vi "Begin.vi"(8 "error in":errorcluster) -> (0 "error out":errorcluster)   [LabVIEW 2015]
doc: "Called before other user functions, this VI is expected to open initial I/O refnums, load in file data, and do all program initialization. Notice that the <B>error out</B> terminal is simply used for data flow. Wiring it to other structures or subVIs ensures that this VI runs first."
uses:
  <vilib>/Rock Robotics/WPI/Camera/WPI_CameraImageSize.ctl
  <vilib>/Rock Robotics/WPI/DriverStation/WPI_DriverStationRobotMode2.ctl
  <vilib>/Rock Robotics/WPI/Joystick/WPI_JoystickDeviceEnum.ctl
  <vilib>/Rock Robotics/WPI/Solenoid/WPI_SolenoidChannel.ctl
  <vilib>/Rock Robotics/SystemInterfaces/AI/FPGA_AIChannel.ctl
  <vilib>/Rock Robotics/WPI/CAN/TalonSRX/WPI_CANTalonSRX_BrakeOverride.ctl
  <vilib>/Rock Robotics/SystemInterfaces/DIO/FPGA_DIOChannel.ctl
  <vilib>/Rock Robotics/SystemInterfaces/DIO/FPGA_DIOPWMChannel.ctl
  <vilib>/Rock Robotics/WPI/CAN/TalonSRX/WPI_CANTalonSRX_APIFeedbackSelect.ctl
  <vilib>/Rock Robotics/WPI/CAN/TalonSRX/WPI_CANTalonSRX_StatusFrame.ctl
  <vilib>/Rock Robotics/WPI/AnalogOutput/WPI_AnalogOutputChannel.ctl
  <vilib>/Rock Robotics/SystemInterfaces/spilib/spi_bus.ctl
  Robot Global Data.vi
  <vilib>/Rock Robotics/WPI/Utilities/WPI_GetSetVariantRefNum.vi
  <vilib>/Rock Robotics/WPI/Solenoid/WPI_SolenoidOpenSingle.vi
  <vilib>/Rock Robotics/WPI/MotorControl/WPI_MotorControlOpenCANTalonSRX.vi
  <vilib>/Rock Robotics/WPI/MotorControl/WPI_MotorControlOpen VictorSP.vi
  <vilib>/Rock Robotics/WPI/Counter/WPI_CounterDigitalInputToDigitalSource.vi
  navX.Library.v2/navX Library v2/IO/Open/Z900_navX_Open_SPI.vi
  <vilib>/Rock Robotics/WPI/CAN/TalonSRX/WPI_CANTalonSRX_APIControlMode.ctl
  <vilib>/Rock Robotics/WPI/Camera/WPI_CameraWhite Balance Values.ctl
  <vilib>/Rock Robotics/WPI/Camera/WPI_CameraExposure Values.ctl
  <vilib>/Rock Robotics/WPI/Ultrasonic/WPI_SonarSRF04DigitalOpen.vi
  <vilib>/Rock Robotics/WPI/Ultrasonic/WPI_SonarSRF04DigitalRefNum Registry Set.vi
  navX-MXP Library/navX-MXP IMU.lvlib
  navX-MXP Library/COMMON/TypeDefs/Value TypeDefs/navX Interface Protocol.ctl
  navX-MXP Library/COMMON/TypeDefs/Value TypeDefs/navX Update Rate.ctl
  <vilib>/Rock Robotics/WPI/Camera/WPI_CameraFrameRate.ctl
  navX.Library.v2/navX Library v2/navX Library v2.lvlib
panel:
  in  "Image Size":T1=enum."320x240"
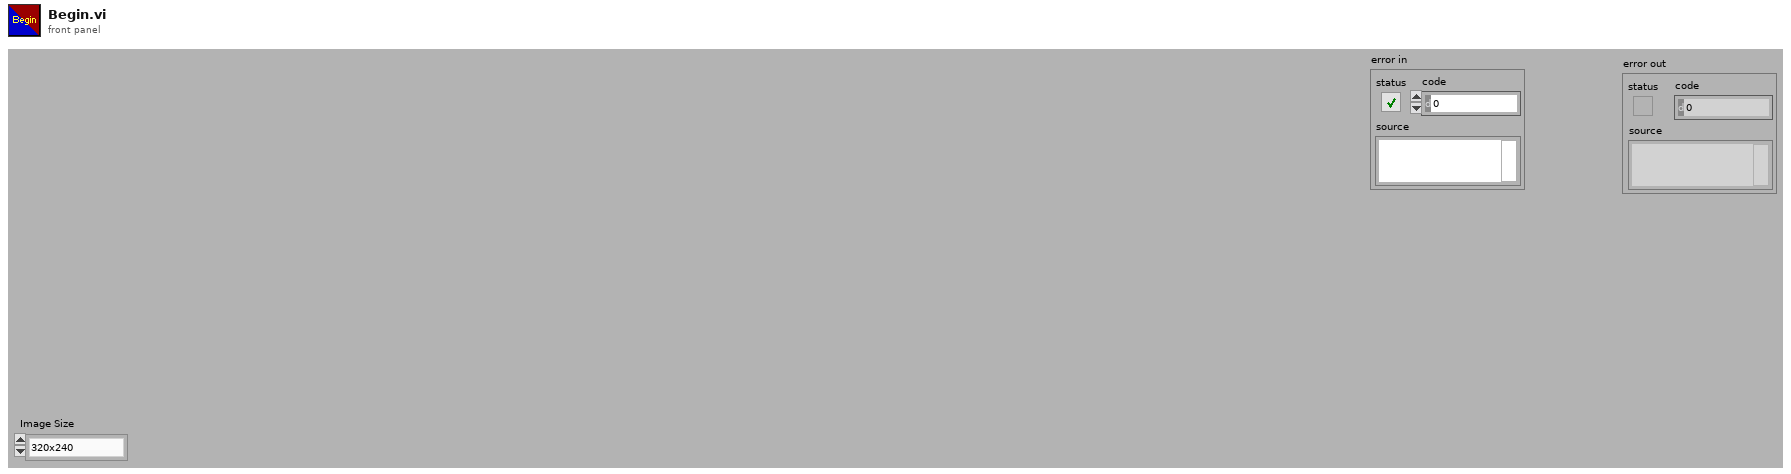
[diagram p1: front panel]
types:
  T1 = typedef "WPI_CameraImageSize.ctl" = enum16{"640x480", "320x240", "160x120", "Custom"}
  T2 = typedef "WPI_AnalogOutputChannel.ctl" = enum8{"AO MXP 0", "AO MXP 1", "Invalid"}
  T3 = typedef "FPGA_AIChannel.ctl" = enum8{"AI 0", "AI 1", "AI 2", "AI 3", "AI MXP 0", "AI MXP 1", "AI MXP 2", "AI MXP 3", "Invalid"}
  T4 = typedef "WPI_CANTalonSRX_StatusFrame.ctl" = enum16{"General Status Frame", "Feedback Status Frame", "Quadrature Status Frame", "Analog Temp Vbat Status Frame", "Pulse Width Status Frame"}
  T5 = typedef "WPI_CANTalonSRX_BrakeOverride.ctl" = enum8{"No Override", "Override to Coast", "Override to Brake"}
  T6 = typedef "WPI_SolenoidChannel.ctl" = enum8{"Solenoid 0", "Solenoid 1", "Solenoid 2", "Solenoid 3", "Solenoid 4", "Solenoid 5", "Solenoid 6", "Solenoid 7", "Invalid"}
  T7 = typedef "WPI_CANTalonSRX_APIFeedbackSelect.ctl" = enum16{"Digital Quadrature Encoder", "Analog Potentiometer", "Analog Encoder", "Count on Quad-A (Rising-Edge)", "Count on Quad-A (Falling-Edge)", "CTR Magnetic Enc (Absolute)", "CTR Magnetic Enc (Relative)", "Pulse Width"}
  T8 = typedef "FPGA_DIOChannel.ctl" = enum8{"DIO 0", "DIO 1", "DIO 2", "DIO 3", "DIO 4", "DIO 5", "DIO 6", "DIO 7", "DIO 8", "DIO 9", "DIO MXP 0", "DIO MXP 1", "DIO MXP 2", "DIO MXP 3", "DIO MXP 4", "DIO MXP 5", "DIO MXP 6", "DIO MXP 7", "DIO MXP 8", "DIO MXP 9", "DIO MXP 10", "DIO MXP 11", "DIO MXP 12", "DIO MXP 13", "DIO MXP 14", "DIO MXP 15", "Invalid"}
  T9 = typedef "FPGA_DIOPWMChannel.ctl" = enum8{"PWM 0", "PWM 1", "PWM 2", "PWM 3", "PWM 4", "PWM 5", "PWM 6", "PWM 7", "PWM 8", "PWM 9", "PWM MXP 0", "PWM MXP 1", "PWM MXP 2", "PWM MXP 3", "PWM MXP 4", "PWM MXP 5", "PWM MXP 6", "PWM MXP 7", "PWM MXP 8", "PWM MXP 9", "Invalid"}
  T10 = typedef "WPI_JoystickDeviceEnum.ctl" = enum16{"USB 0", "USB 1", "USB 2", "USB 3", "USB 4", "USB 5"}
  T11 = typedef "WPI_DriverStationRobotMode2.ctl" = enum16{"Autonomous Disabled", "Autonomous Enabled", "Teleop Disabled", "Teleop Enabled", "Disconnected", "Finish", "Test Disabled", "Test Enabled", "Emergency Stopped"}
  T12 = typedef "navX-MXP IMU.lvlib/navX Update Rate.ctl" = u8
  T13 = typedef "navX-MXP IMU.lvlib/navX Interface Protocol.ctl" = enum16{"SPI", "I2C"}
  T14 = typedef "spi_bus.ctl" = enum16{"SPI On-Board, CS0", "SPI On-Board, CS1", "SPI On-Board, CS2", "SPI On-Board, CS3", "SPI MXP", "Invalid"}
  T15 = typedef "navX-MXP IMU.lvlib/navX Device TypeDef.ctl" = cluster{"navX Interface Protocol":T13, "navX Interface Protocol TypeDefs":cluster{"SPIDevRef":T16, "I2CDevRef":T17}, "navX System Information":cluster{"Board Information":T19, "Status":T20, "Offsets":T24}, "navX Common Information":cluster{"Update Rate (4Hz-60Hz)":T12, "refnum name":string, "error":errorcluster}}
  T16 = typedef "WPI_SPIDevRef.ctl" = cluster{"DevStatus":errorcluster, "Handle":i32, "SPI Bus":T14}
  T17 = typedef "WPI_I2CDevRef.ctl" = cluster{"DevStatus":errorcluster, "Device Address":u8, "Handle":i32, "I2C Bus":T18}
  T18 = typedef "i2c_bus.ctl" = enum16{"I2C On-Board", "I2C MXP", "Invalid"}
  T19 = typedef "navX-MXP IMU.lvlib/navX Board Information.ctl" = cluster{"WhoAmI (50 | 0x32)":u8, "Board Revision":u8, "Firmware Major Version":u8, "Firmware Minor Version":u8}
  T20 = typedef "navX-MXP IMU.lvlib/navX Status Data.ctl" = cluster{"Update Rate Hz":u8, "Accelerometer Full-Scale Range":u8, "Gyro Full-Scale Range":u16, "NAVX_OP_STATUS":T21, "NAVX_CAL_STATUS":T22, "NAVX_SELFTEST_STATUS":u8, "NAVX_SENSOR_STATUS":T23}
  T21 = typedef "navX-MXP IMU.lvlib/navX NAVX_OP_STATUS.ctl" = u8
  T22 = typedef "navX-MXP IMU.lvlib/navX NAVX_CAL_STATUS.ctl" = u8
  T23 = typedef "navX-MXP IMU.lvlib/navX NAVX_SENSOR_STATUS.ctl" = cluster{"MOVING":bool, "YAW_STABLE":bool, "MAG_DISTURBANCE":bool, "ALTITUDE_VALID":bool, "SEALEVEL_PRESS_SET":bool, "FUSED_HEADING_VALID":bool}
  T24 = typedef "navX-MXP IMU.lvlib/navX Offsets Data.ctl" = cluster{"Yaw":dbl, "Quat W":dbl, "Quat X":dbl, "Quat Y":dbl, "Quat Z":dbl}
  T25 = typedef "navX Library v2.lvlib/Z900_navX_DeviceTypeDef.ctl" = cluster{"Interface":cluster{"Protocol":T26, "Update Rate (4Hz-60Hz)":u8, "navX Open TypeDef":variant}, "Notify Packet":refnum<notifier>, "Loop VI Refnum":refnum<vi>, "Ready to Close Occurrence Refnum":refnum<k4>}
  T26 = typedef "navX Library v2.lvlib/Z900_navX_ProtocolTypeDef.ctl" = enum16{"SERIAL", "I2C", "SPI"}
  T27 = typedef "WPI_CameraExposure Values.ctl" = enum16{"Auto", "Flicker-free 50 Hz", "Flicker-free 60 Hz", "Hold current", "Custom"}
  T28 = typedef "WPI_CameraWhite Balance Values.ctl" = enum16{"Auto", "Fixed indoor", "Fixed outdoor 1", "Fixed outdoor 2", "Fixed fluorescent 1", "Fixed fluorescent 2", "Hold current", "Custom"}
  T29 = typedef "WPI_CameraFrameRate.ctl" = u32
  T30 = typedef "WPI_CameraDevRef.ctl" = cluster{"Camera Address":string, "CameraStatus":errorcluster}
  T31 = typedef "WPI_DigitalInputDevRef.ctl" = cluster{"DevStatus":errorcluster, "DIO Channel":T8}
  T32 = typedef "FPGA_CounterEncoderSourceConvertionLVSourceType.ctl" = cluster{"DevStatus":errorcluster, "AnalogTriggerMode?":bool, "DigitalMode":cluster{"DIO Channel":T33}, "AnalogTriggerMode":cluster{"AnalogTriggerIndex":T34, "OutputType":T35}}
  T33 = typedef "FPGA_DIODigitalSourceChannel.ctl" = enum8{"DIO 0", "DIO 1", "DIO 2", "DIO 3", "DIO 4", "DIO 5", "DIO 6", "DIO 7", "DIO 8", "DIO 9", "DIO MXP 0", "DIO MXP 1", "DIO MXP 2", "DIO MXP 3", "DIO MXP 4", "DIO MXP 5", "DIO MXP 6", "DIO MXP 7", "DIO MXP 8", "DIO MXP 9", "DIO MXP 10", "DIO MXP 11", "DIO MXP 12", "DIO MXP 13", "DIO MXP 14", "DIO MXP 15", "Disabled"}
  T34 = typedef "FPGA_AnalogTriggerIndex.ctl" = enum8{"Trig 0", "Trig 1", "Trig 2", "Trig 3", "Trig 4", "Trig 5", "Trig 6", "Trig 7", "Invalid"}
  T35 = typedef "FPGA_AnalogTriggerOutType.ctl" = enum16{"InWindow", "TriggerState", "Rising", "Falling"}
  T36 = typedef "WPI_EncoderDevRef.ctl" = cluster{"DevStatus":errorcluster, "EncoderIndex":T37, "CounterIndex":T38, "DistancePerCount":dbl, "Decoding Type":T39}
  T37 = typedef "FPGA_EncoderIdx.ctl" = enum8{"Enc 0", "Enc 1", "Enc 2", "Enc 3", "Enc 4", "Enc 5", "Enc 6", "Enc 7", "Invalid"}
  T38 = typedef "FPGA_CounterCtrSystemIndex.ctl" = enum8{"Ctr 0", "Ctr 1", "Ctr 2", "Ctr 3", "Ctr 4", "Ctr 5", "Ctr 6", "Ctr 7", "Invalid"}
  T39 = typedef "WPI_EncoderType.ctl" = enum16{"1x", "2x", "4x"}
  T40 = typedef "WPI_UltrasonicDeviceRef.ctl" = cluster{"DevStatus":errorcluster, "Ping Channel":T8, "Echo Channel":T8, "CntIndex":T38}
  T41 = typedef "WPI_CompressorDevRef.ctl" = cluster{"DevStatus":errorcluster, "Pneumatics Control Module":u8}
  T42 = typedef "WPI_JoystickDevRef.ctl" = cluster{"Device":T10}
  T43 = typedef "WPI_SolenoidDevRef.ctl" = cluster{"DevStatus":errorcluster, "Pneumatics Control Module":u8, "Forward Solenoid Channel":T6, "Reverse Solenoid Channel":T6}
  T44 = typedef "WPI_MotorControlDeviceRef.ctl" = cluster{"DeviceStatus":errorcluster, "Type":T45, "PWM":cluster{"PWM Channel":T9, "DeadBand":T46}, "CAN":cluster{"Device Number":u8, "Control Mode":T47, "Semaphore":T48, "Max Vout":dbl, "TalonSRX Control Mode":T49}, "Invert":bool}
  T45 = typedef "WPI_MotorControlType.ctl" = enum16{"PWM", "CAN", "CANTalonSRX"}
  T46 = typedef "WPI_PWMDeadband.ctl" = cluster{"Name":string, "maxPositivePwm":i32, "minPositivePwm":i32, "centerPwm":i32, "maxNegativePwm":i32, "minNegativePwm":i32, "angularRange":u16}
  T47 = typedef "WPI_CANJaguar_ControlMode.ctl" = enum8{"Percent VBus", "Current", "Speed", "Position", "Voltage"}
  T48 = typedef "Semaphore RefNum" = refnum<k1>
  T49 = typedef "WPI_CANTalonSRX_APIControlMode.ctl" = enum8{"Percent VBus", "Speed", "Position", "Slave", "Unchanged / Invalid", "Voltage Compensation", "Current", "Motion Profile"}
  T50 = typedef "WPI_AnalogChannelDevRef.ctl" = cluster{"DevStatus":errorcluster, "Analog Channel":T3}
  T51 = typedef "WPI_ServoDeviceRef.ctl" = cluster{"DeviceStatus":errorcluster, "PWM Channel":T9, "DeadBand":T46}
  T52 = typedef "WPI_AOChannelDevRef.ctl" = cluster{"DevStatus":errorcluster, "AO Channel":T2}
  T53 = typedef "WPI_DigitalOutputDevRef.ctl" = cluster{"DIO Channel":T8, "DevStatus":errorcluster}
  T54 = typedef "WPI_PotentiometerDevRef.ctl" = cluster{"DevStatus":errorcluster, "Analog Channel":T3, "Invert Output":bool}
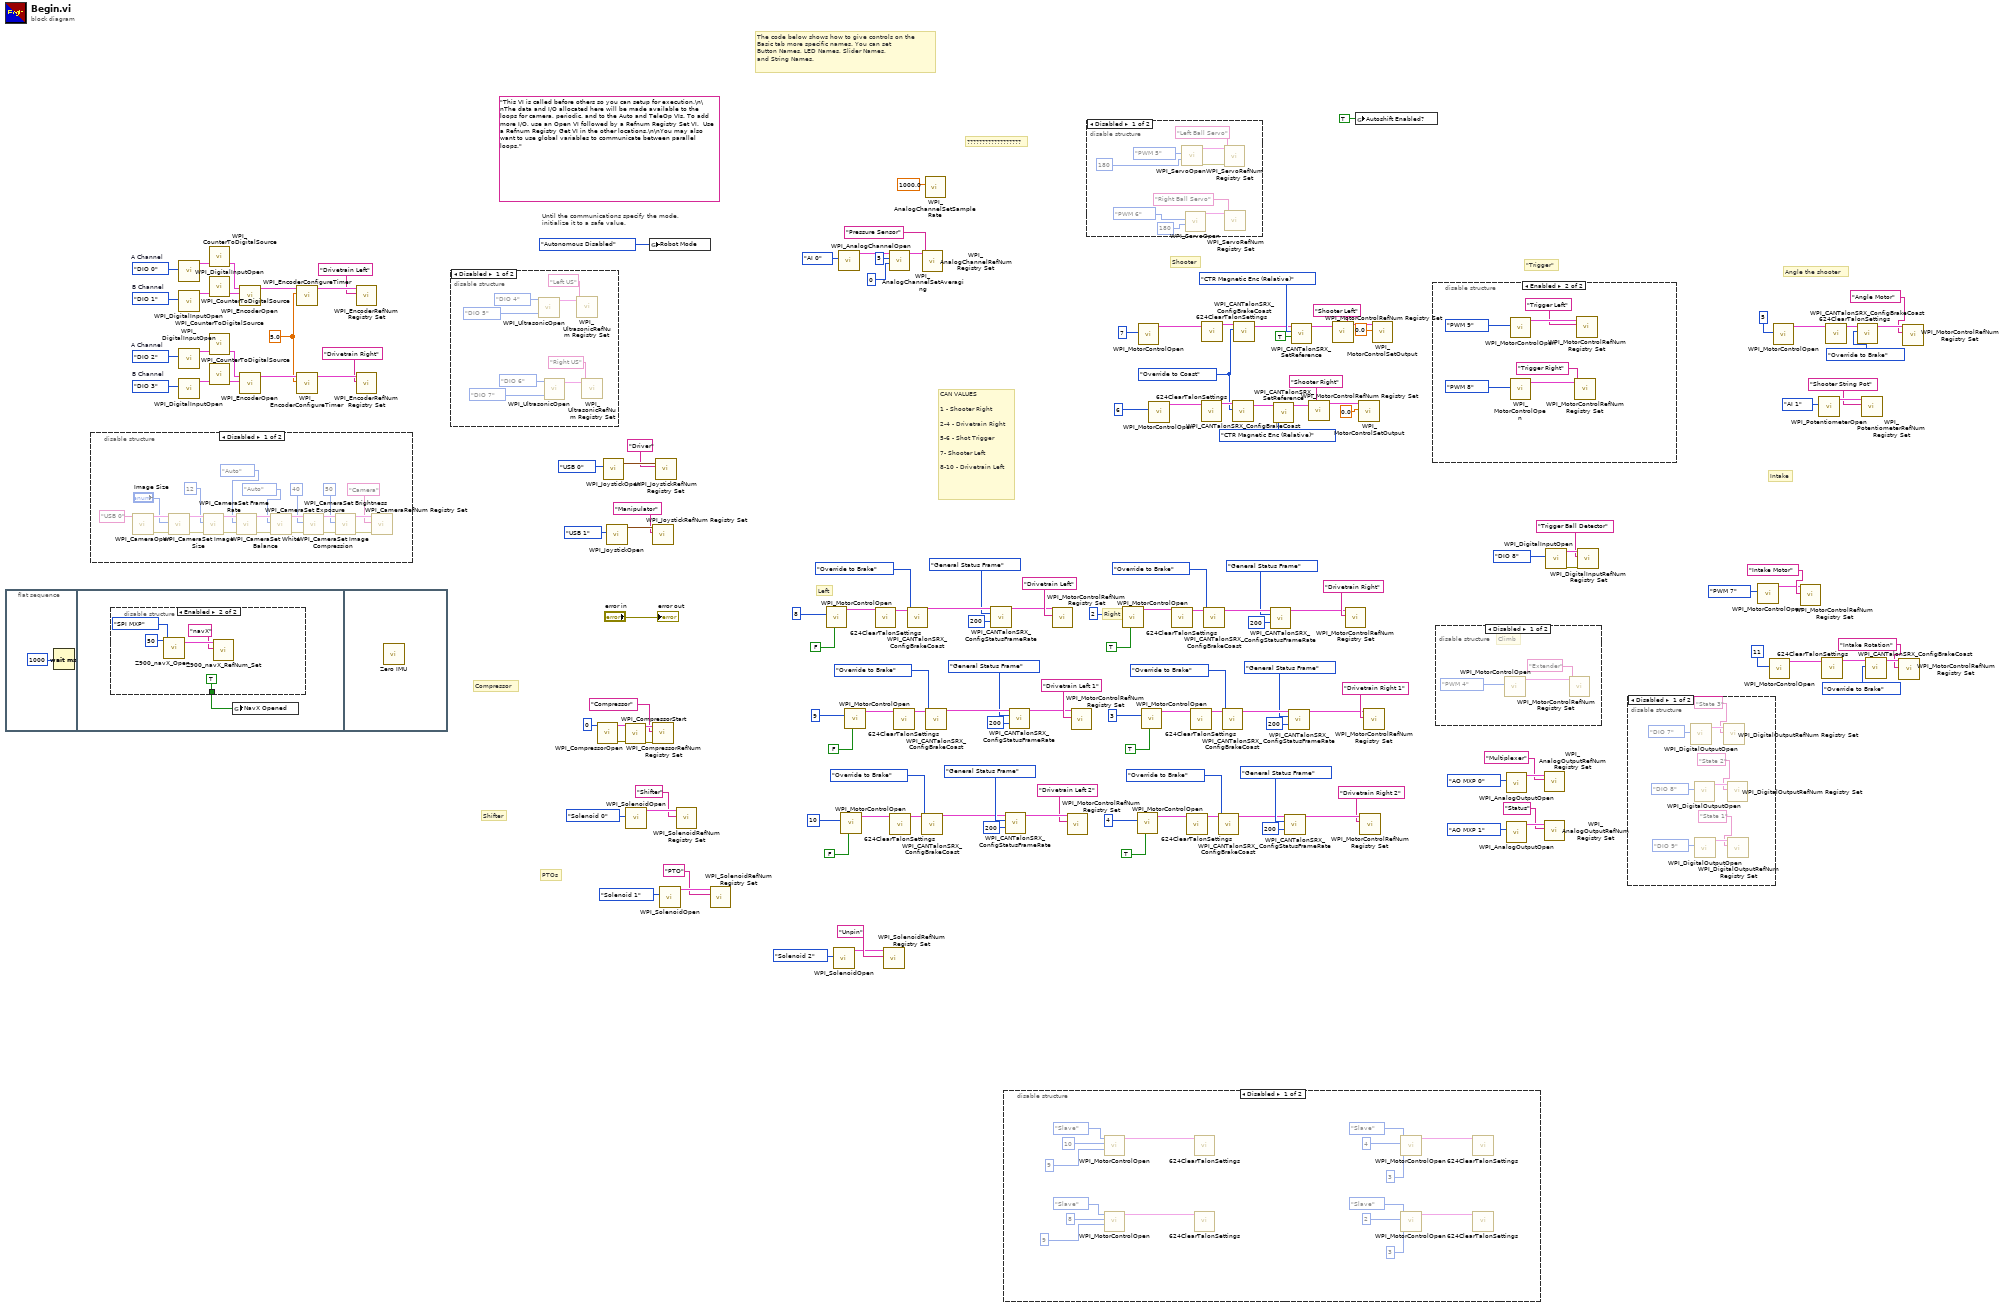
[diagram p0: block diagram]
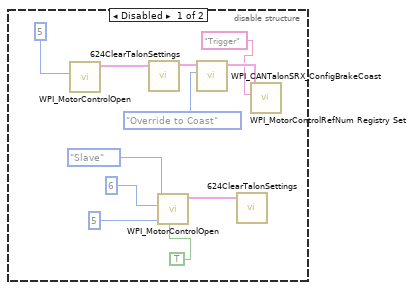
[diagram p8: hidden frame]
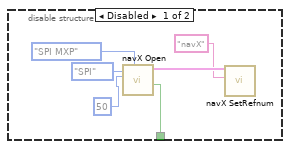
[diagram p9: hidden frame]
diagram:
  w78 = FPGA_DIOChannel."DIO 3"  # B Channel
  w81 = FPGA_DIOChannel."DIO 0"  # A Channel
  w84 = FPGA_DIOChannel."DIO 1"  # B Channel
  w89 = 5.0 ("Minimum Rate")
  w92 = FPGA_DIOChannel."DIO 2"  # A Channel
  w108 = WPI_CANTalonSRX_BrakeOverride."Override to Coast" ("Brake / Coast Mode")
  (unwired) "This VI is called before others so you can setup for execution.\n\nThe data and I/O allocated here will be made available to the loops for camera, periodic, and to the Auto and TeleOp VIs. To add more I/O, use an Open VI followed by a Refnum Registry Set VI.  Use a Refnum Registry Get VI in the other locations.\n\nYou may also want to use global variables to communicate between parallel loops."
  # "??????????????????"
  # "CAN VALUES\n\n1 - Shooter Right\n\n2-4 - Drivetrain Right\n\n5-6 - Shot Trigger\n\n7- Shooter Left\n\n8-10 - Drivetrain Left"
  # "Angle the shooter"
  # "PTOs"
  # "Intake"
  # "\"Trigger\""
  # "Shooter"
  # "Left"
  # "Right"
  # "Shifter"
  # "Compressor"
  # "The code below shows how to give controls on the\nBasic tab more specific names. You can set\nButton Names, LED Names, Slider Names,\nand String Names."
  # "Until the communications specify the mode,\ninitialize it to a safe value."
  n1 = flat-sequence {
    frame #0 {
      n2 = Wait (ms)(milliseconds to wait=u32 1000) -> ()  [unwired: 1 out]
    }
    frame #1 {
      n3 = disable-structure shown="Enabled" {
        disable-tunnel: [w161 TRUE ("NavX Opened")] -> w160
        frame Disabled {
          n4 = call "navX Open.vi"("SPI Bus"=spi_bus."SPI MXP", "Update Rate (4Hz-60Hz)"=T12 50, "navX Interface Protocol"=navX_Interface_Protocol."SPI") -> ("Opened?"=w161:bool, "navX Device TypeDef"=w166:T15)  [unwired: 6 in, 1 out]
          n5 = call "navX SetRefnum.vi"("refnum name"="navX", "navX Device TypeDef"=w166) -> ()  [unwired: 8 in, 2 out]
        }
        frame Enabled {
          n6 = call-poly "Z900_navX_Open.vi"("SPI Bus"=spi_bus."SPI MXP", "Update Rate (4Hz-60Hz)"=u8 50) -> ("navX Device"=w171:T25)  [unwired: 8 in, 1 out]
          n7 = call "Z900_navX_RefNum_Set.vi"("refnum name"="navX", "navX Device"=w171) -> ()  [unwired: 8 in, 2 out]
        }
      }
      n8 = global write "Robot Global Data.vi" "NavX Opened"(w160) -> ()
    }
    frame #2 {
      n9 = call "Zero IMU.vi"() -> ()  [unwired: 12 in]
    }
  }
  n10 = disable-structure shown="Disabled" {
    frame Disabled {
      n11 = call <vilib>:"WPI_CameraOpen.vi"("Camera Address"="USB 0" ("format string")) -> ("error out"=w181:errorcluster, "CameraDevRef"=w180:T30)  [unwired: 1 in, 8 out]
      n12 = call <vilib>:"WPI_CameraSet Image Size.vi"("error in (no error)"=w181, "Image Size"="Image Size", "CameraDevRef"=w180) -> ("error out"=w183:errorcluster, "CameraDevRef Out"=w182:T30)  [unwired: 1 in, 6 out]
      n13 = call <vilib>:"WPI_CameraSet Frame Rate.vi"("error in (no error)"=w183, "Frame Rate (fps)"=T29 12, "CameraDevRef"=w182) -> ("error out"=w185:errorcluster, "CameraDevRef Out"=w184:T30)  [unwired: 7 out]
      n14 = call <vilib>:"WPI_CameraSet White Balance.vi"("error in (no error)"=w185, "White Balance"=WPI_CameraWhite_Balance_Values."Auto", "CameraDevRef"=w184) -> ("error out"=w187:errorcluster, "CameraDevRef Out"=w186:T30)  [unwired: 1 in, 6 out]
      n15 = call <vilib>:"WPI_CameraSet Exposure.vi"("error in (no error)"=w187, "Exposure"=WPI_CameraExposure_Values."Auto", "CameraDevRef"=w186) -> ("error out"=w189:errorcluster, "CameraDevRef Out"=w188:T30)  [unwired: 1 in, 6 out]
      n16 = call <vilib>:"WPI_CameraSet Image Compression.vi"("error in (no error)"=w189, "Compression"=40, "CameraDevRef"=w188) -> ("error out"=w191:errorcluster, "CameraDevRef Out"=w190:T30)  [unwired: 7 out]
      n17 = call <vilib>:"WPI_CameraSet Brightness.vi"("error in (no error)"=w191, "Brightness"=50, "CameraDevRef"=w190) -> ("error out"=w193:errorcluster, "CameraDevRef Out"=w192:T30)  [unwired: 7 out]
      n18 = call <vilib>:"WPI_CameraRefNum Registry Set.vi"("error in (no error)"=w193, "refnum name"="Camera", "CameraDevRef"=w192) -> ()  [unwired: 1 in, 8 out]
    }
    frame Enabled {
    }
  }
  n19 = call <vilib>:"WPI_DigitalInputOpen.vi"("DIO Channel"=w81) -> ("DigitalInputDevRef"=w82:T31)  [unwired: 1 in, 9 out]
  n20 = call <vilib>:"WPI_DigitalInputOpen.vi"("DIO Channel"=w84) -> ("DigitalInputDevRef"=w85:T31)  [unwired: 1 in, 9 out]
  n21 = call <vilib>:"WPI_DigitalInputOpen.vi"("DIO Channel"=w92) -> ("DigitalInputDevRef"=w93:T31)  [unwired: 1 in, 9 out]
  n22 = call <vilib>:"WPI_DigitalInputOpen.vi"("DIO Channel"=w78) -> ("DigitalInputDevRef"=w90:T31)  [unwired: 1 in, 9 out]
  n23 = call-poly <vilib>:"WPI_CounterToDigitalSource.vi"("DigitalInputDevRef"=w82) -> ("Digital Source"=w83:T32)  [unwired: 6 out]
  n24 = call-poly <vilib>:"WPI_CounterToDigitalSource.vi"("DigitalInputDevRef"=w85) -> ("Digital Source"=w86:T32)  [unwired: 6 out]
  n25 = call-poly <vilib>:"WPI_CounterToDigitalSource.vi"("DigitalInputDevRef"=w93) -> ("Digital Source"=w94:T32)  [unwired: 6 out]
  n26 = call-poly <vilib>:"WPI_CounterToDigitalSource.vi"("DigitalInputDevRef"=w90) -> ("Digital Source"=w91:T32)  [unwired: 6 out]
  n27 = call <vilib>:"WPI_EncoderOpen.vi"("BSource"=w86, "ASource"=w83) -> ("EncoderDevRef"=w87:T36)  [unwired: 6 in, 3 out]
  n28 = call <vilib>:"WPI_EncoderOpen.vi"("BSource"=w91, "ASource"=w94) -> ("EncoderDevRef"=w95:T36)  [unwired: 6 in, 3 out]
  n29 = call <vilib>:"WPI_EncoderConfigureTimer.vi"("Minimum Rate"=w89, "EncoderDevRef"=w87) -> ("EncoderDevRef"=w88:T36)  [unwired: 8 in, 1 out]
  n30 = call <vilib>:"WPI_EncoderConfigureTimer.vi"("Minimum Rate"=w89, "EncoderDevRef"=w95) -> ("EncoderDevRef"=w96:T36)  [unwired: 8 in, 1 out]
  n31 = call <vilib>:"WPI_EncoderRefNum Registry Set.vi"("refnum name"="Drivetrain Left", "EncoderDevRef"=w88) -> ()  [unwired: 8 in, 2 out]
  n32 = call <vilib>:"WPI_EncoderRefNum Registry Set.vi"("refnum name"="Drivetrain Right", "EncoderDevRef"=w96) -> ()  [unwired: 8 in, 2 out]
  n33 = disable-structure shown="Disabled" {
    frame Disabled {
      n34 = call-poly <vilib>:"WPI_UltrasonicOpen.vi"("Echo DIO Channel"=FPGA_DIOChannel."DIO 5", "Ping DIO Channel"=FPGA_DIOChannel."DIO 4") -> ("SonarSRF04DevRef"=w201:T40)  [unwired: 8 in, 1 out]
      n35 = call-poly <vilib>:"WPI_UltrasonicOpen.vi"("Echo DIO Channel"=FPGA_DIOChannel."DIO 7", "Ping DIO Channel"=FPGA_DIOChannel."DIO 6") -> ("SonarSRF04DevRef"=w194:T40)  [unwired: 8 in, 1 out]
      n36 = call-poly <vilib>:"WPI_UltrasonicRefNum Registry Set.vi"("refnum name"="Left US", "SonarSRF04DevRef"=w201) -> ()  [unwired: 8 in, 2 out]
      n37 = call-poly <vilib>:"WPI_UltrasonicRefNum Registry Set.vi"("refnum name"="Right US", "SonarSRF04DevRef"=w194) -> ()  [unwired: 8 in, 2 out]
    }
    frame Enabled {
    }
  }
  n38 = call <vilib>:"WPI_CompressorOpen.vi"("Pneumatics Control Module (0)"=0) -> ("CompressorDevRef"=w153:T41, "error out"=w150:errorcluster)  [unwired: 13 in]
  n39 = call <vilib>:"WPI_JoystickOpen.vi"("JoystickDevice"=WPI_JoystickDeviceEnum."USB 0") -> ("JoystickDevRef"=w157:T42)  [unwired: 10 in]
  n40 = call <vilib>:"WPI_JoystickOpen.vi"("JoystickDevice"=WPI_JoystickDeviceEnum."USB 1") -> ("JoystickDevRef"=w135:T42)  [unwired: 10 in]
  n41 = call <vilib>:"WPI_CompressorStart.vi"("error in (no error)"=w150, "CompressorDevRef"=w153) -> ("error out"=w149:errorcluster, "CompressorDevRef"=w152:T41)  [unwired: 8 in]
  n42 = call-poly <vilib>:"WPI_SolenoidOpen.vi"("Solenoid Channel"=WPI_SolenoidChannel."Solenoid 0") -> ("SolenoidDevRef"=w147:T43)  [unwired: 9 in, 1 out]
  n43 = global write "Robot Global Data.vi" "Robot Mode"(WPI_DriverStationRobotMode2."Autonomous Disabled" ("Robot Mode")) -> ()
  n44 = call <vilib>:"WPI_JoystickRefNum Registry Set.vi"("refnum name"="Manipulator", "JoystickDevRef"=w135) -> ()  [unwired: 8 in, 2 out]
  n45 = call <vilib>:"WPI_CompressorRefNum Registry Set.vi"("error in (no error)"=w149, "refnum name"="Compressor", "CompressorDevRef"=w152) -> ()  [unwired: 7 in, 2 out]
  n46 = call <vilib>:"WPI_JoystickRefNum Registry Set.vi"("refnum name"="Driver", "JoystickDevRef"=w157) -> ()  [unwired: 8 in, 2 out]
  n47 = call-poly <vilib>:"WPI_SolenoidOpen.vi"("Solenoid Channel"=WPI_SolenoidChannel."Solenoid 1") -> ("SolenoidDevRef"=w114:T43)  [unwired: 9 in, 1 out]
  n48 = call <vilib>:"WPI_SolenoidRefNum Registry Set.vi"("refnum name"="Shifter", "SolenoidDevRef"=w147) -> ()  [unwired: 8 in, 2 out]
  n49 = call <vilib>:"WPI_SolenoidRefNum Registry Set.vi"("refnum name"="PTO", "SolenoidDevRef"=w114) -> ()  [unwired: 8 in, 2 out]
  n50 = call-poly <vilib>:"WPI_MotorControlOpen.vi"("Invert"=FALSE, "Device Number"=8) -> ("MotorControlDeviceRef"=w30:T44)  [unwired: 8 in, 1 out]
  n51 = call-poly <vilib>:"WPI_SolenoidOpen.vi"("Solenoid Channel"=WPI_SolenoidChannel."Solenoid 2") -> ("SolenoidDevRef"=w60:T43)  [unwired: 9 in, 1 out]
  n52 = call <vilib>:"WPI_AnalogChannelOpen.vi"("Analog Channel"=FPGA_AIChannel."AI 0") -> ("AIDeviceRef"=w16:T50)  [unwired: 9 in, 1 out]
  n53 = call-poly <vilib>:"WPI_MotorControlOpen.vi"("Invert"=FALSE, "Device Number"=10) -> ("MotorControlDeviceRef"=w43:T44)  [unwired: 8 in, 1 out]
  n54 = call-poly <vilib>:"WPI_MotorControlOpen.vi"("Invert"=FALSE, "Device Number"=9) -> ("MotorControlDeviceRef"=w139:T44)  [unwired: 8 in, 1 out]
  n55 = call "624ClearTalonSettings.vi"("CAN Talon SRX Ref Out"=w30) -> ("CAN Talon SRX Ref Out 2"=w31:T44)  [unwired: 10 in]
  n56 = call <vilib>:"WPI_SolenoidRefNum Registry Set.vi"("refnum name"="Unpin", "SolenoidDevRef"=w60) -> ()  [unwired: 8 in, 2 out]
  n57 = call <vilib>:"WPI_AnalogChannelSetAveraging.vi"("OversampleBits"=u8 0, "AverageBits"=u8 5, "AIDeviceRef"=w16) -> ("AIDeviceRef"=w15:T50)  [unwired: 7 in, 1 out]
  n58 = call "624ClearTalonSettings.vi"("CAN Talon SRX Ref Out"=w43) -> ("CAN Talon SRX Ref Out 2"=w42:T44)  [unwired: 10 in]
  n59 = call "624ClearTalonSettings.vi"("CAN Talon SRX Ref Out"=w139) -> ("CAN Talon SRX Ref Out 2"=w140:T44)  [unwired: 10 in]
  n60 = call <vilib>:"WPI_CANTalonSRX_ConfigBrakeCoast.vi"("Brake / Coast Mode"=WPI_CANTalonSRX_BrakeOverride."Override to Brake", "CAN Talon SRX Ref"=w31) -> ("CAN Talon SRX Ref"=w23:T44)  [unwired: 8 in, 1 out]
  n61 = call <vilib>:"WPI_CANTalonSRX_ConfigBrakeCoast.vi"("Brake / Coast Mode"=WPI_CANTalonSRX_BrakeOverride."Override to Brake", "CAN Talon SRX Ref"=w42) -> ("CAN Talon SRX Ref"=w50:T44)  [unwired: 8 in, 1 out]
  n62 = call <vilib>:"WPI_AnalogChannelRefNum Registry Set.vi"("refnum name"="Pressure Sensor", "AIDeviceRef"=w15) -> ()  [unwired: 8 in, 2 out]
  n63 = call <vilib>:"WPI_AnalogChannelSetSampleRate.vi"("Samples Per Second (per channel)"=1000.0) -> ()  [unwired: 10 in, 1 out]
  n64 = call <vilib>:"WPI_CANTalonSRX_ConfigBrakeCoast.vi"("Brake / Coast Mode"=WPI_CANTalonSRX_BrakeOverride."Override to Brake", "CAN Talon SRX Ref"=w140) -> ("CAN Talon SRX Ref"=w64:T44)  [unwired: 8 in, 1 out]
  n65 = call <vilib>:"WPI_CANTalonSRX_ConfigStatusFrameRate.vi"("CAN Talon SRX Ref"=w23, "Talon SRX Status Frame"=WPI_CANTalonSRX_StatusFrame."General Status Frame", "Frame Rate Ms"=u32 200) -> ("CAN Talon SRX Ref"=w22:T44)  [unwired: 12 in]
  n66 = disable-structure shown="Disabled" {
    frame Disabled {
      n67 = call-poly <vilib>:"WPI_MotorControlOpen.vi"("Master Device Number"=u8 9, "Device Number"=u8 10, "Control Mode"=WPI_CANTalonSRX_APIControlMode."Slave") -> ("MotorControlDeviceRef"=w209:T44)  [unwired: 7 in, 1 out]
      n68 = call-poly <vilib>:"WPI_MotorControlOpen.vi"("Master Device Number"=u8 9, "Device Number"=u8 8, "Control Mode"=WPI_CANTalonSRX_APIControlMode."Slave") -> ("MotorControlDeviceRef"=w210:T44)  [unwired: 7 in, 1 out]
      n69 = call "624ClearTalonSettings.vi"("CAN Talon SRX Ref Out"=w209) -> ()  [unwired: 10 in, 1 out]
      n70 = call "624ClearTalonSettings.vi"("CAN Talon SRX Ref Out"=w210) -> ()  [unwired: 10 in, 1 out]
      n71 = call-poly <vilib>:"WPI_MotorControlOpen.vi"("Master Device Number"=u8 3, "Device Number"=u8 4, "Control Mode"=WPI_CANTalonSRX_APIControlMode."Slave") -> ("MotorControlDeviceRef"=w202:T44)  [unwired: 7 in, 1 out]
      n72 = call-poly <vilib>:"WPI_MotorControlOpen.vi"("Master Device Number"=u8 3, "Device Number"=u8 2, "Control Mode"=WPI_CANTalonSRX_APIControlMode."Slave") -> ("MotorControlDeviceRef"=w217:T44)  [unwired: 7 in, 1 out]
      n73 = call "624ClearTalonSettings.vi"("CAN Talon SRX Ref Out"=w202) -> ()  [unwired: 10 in, 1 out]
      n74 = call "624ClearTalonSettings.vi"("CAN Talon SRX Ref Out"=w217) -> ()  [unwired: 10 in, 1 out]
    }
    frame Enabled {
    }
  }
  n75 = call <vilib>:"WPI_CANTalonSRX_ConfigStatusFrameRate.vi"("CAN Talon SRX Ref"=w50, "Talon SRX Status Frame"=WPI_CANTalonSRX_StatusFrame."General Status Frame", "Frame Rate Ms"=u32 200) -> ("CAN Talon SRX Ref"=w51:T44)  [unwired: 12 in]
  n76 = call <vilib>:"WPI_CANTalonSRX_ConfigStatusFrameRate.vi"("CAN Talon SRX Ref"=w64, "Talon SRX Status Frame"=WPI_CANTalonSRX_StatusFrame."General Status Frame", "Frame Rate Ms"=u32 200) -> ("CAN Talon SRX Ref"=w63:T44)  [unwired: 12 in]
  n77 = call <vilib>:"WPI_MotorControlRefNum Registry Set.vi"("refnum name"="Drivetrain Left", "MotorControlDevRef"=w22) -> ()  [unwired: 8 in, 2 out]
  n78 = call <vilib>:"WPI_MotorControlRefNum Registry Set.vi"("refnum name"="Drivetrain Left 2", "MotorControlDevRef"=w51) -> ()  [unwired: 8 in, 2 out]
  n79 = call <vilib>:"WPI_MotorControlRefNum Registry Set.vi"("refnum name"="Drivetrain Left 1", "MotorControlDevRef"=w63) -> ()  [unwired: 8 in, 2 out]
  n80 = disable-structure shown="Disabled" {
    frame Disabled {
      n81 = call <vilib>:"WPI_ServoOpen.vi"("Angular Range"=u16 180, "PWM Channel"=FPGA_DIOPWMChannel."PWM 5") -> ("error out"=w224:errorcluster, "ServoDeviceRef"=w223:T51)  [unwired: 8 in]
      n82 = call <vilib>:"WPI_ServoOpen.vi"("Angular Range"=u16 180, "PWM Channel"=FPGA_DIOPWMChannel."PWM 6") -> ("ServoDeviceRef"=w222:T51)  [unwired: 8 in, 1 out]
      n83 = call <vilib>:"WPI_ServoRefNum Registry Set.vi"("error in (no error)"=w224, "refnum name"="Left Ball Servo", "ServoDeviceRef"=w223) -> ()  [unwired: 7 in, 2 out]
      n84 = call <vilib>:"WPI_ServoRefNum Registry Set.vi"("refnum name"="Right Ball Servo", "ServoDeviceRef"=w222) -> ()  [unwired: 8 in, 2 out]
    }
    frame Enabled {
    }
  }
  n85 = call-poly <vilib>:"WPI_MotorControlOpen.vi"("Invert"=TRUE, "Device Number"=2) -> ("MotorControlDeviceRef"=w33:T44)  [unwired: 8 in, 1 out]
  n86 = call-poly <vilib>:"WPI_MotorControlOpen.vi"("Invert"=TRUE, "Device Number"=4) -> ("MotorControlDeviceRef"=w40:T44)  [unwired: 8 in, 1 out]
  n87 = call-poly <vilib>:"WPI_MotorControlOpen.vi"("Device Number"=u8 7) -> ("MotorControlDeviceRef"=w106:T44)  [unwired: 9 in, 1 out]
  n88 = call-poly <vilib>:"WPI_MotorControlOpen.vi"("Invert"=TRUE, "Device Number"=3) -> ("MotorControlDeviceRef"=w142:T44)  [unwired: 8 in, 1 out]
  n89 = call-poly <vilib>:"WPI_MotorControlOpen.vi"("Device Number"=u8 6) -> ("MotorControlDeviceRef"=w110:T44)  [unwired: 9 in, 1 out]
  n90 = call "624ClearTalonSettings.vi"("CAN Talon SRX Ref Out"=w33) -> ("CAN Talon SRX Ref Out 2"=w32:T44)  [unwired: 10 in]
  n91 = call "624ClearTalonSettings.vi"("CAN Talon SRX Ref Out"=w40) -> ("CAN Talon SRX Ref Out 2"=w41:T44)  [unwired: 10 in]
  n92 = call "624ClearTalonSettings.vi"("CAN Talon SRX Ref Out"=w142) -> ("CAN Talon SRX Ref Out 2"=w141:T44)  [unwired: 10 in]
  n93 = call "624ClearTalonSettings.vi"("CAN Talon SRX Ref Out"=w110) -> ("CAN Talon SRX Ref Out 2"=w111:T44)  [unwired: 10 in]
  n94 = call "624ClearTalonSettings.vi"("CAN Talon SRX Ref Out"=w106) -> ("CAN Talon SRX Ref Out 2"=w107:T44)  [unwired: 10 in]
  n95 = call <vilib>:"WPI_CANTalonSRX_ConfigBrakeCoast.vi"("Brake / Coast Mode"=WPI_CANTalonSRX_BrakeOverride."Override to Brake", "CAN Talon SRX Ref"=w32) -> ("CAN Talon SRX Ref"=w25:T44)  [unwired: 8 in, 1 out]
  n96 = call <vilib>:"WPI_CANTalonSRX_ConfigBrakeCoast.vi"("Brake / Coast Mode"=WPI_CANTalonSRX_BrakeOverride."Override to Brake", "CAN Talon SRX Ref"=w41) -> ("CAN Talon SRX Ref"=w48:T44)  [unwired: 8 in, 1 out]
  n97 = call <vilib>:"WPI_CANTalonSRX_ConfigBrakeCoast.vi"("Brake / Coast Mode"=WPI_CANTalonSRX_BrakeOverride."Override to Brake", "CAN Talon SRX Ref"=w141) -> ("CAN Talon SRX Ref"=w66:T44)  [unwired: 8 in, 1 out]
  n98 = call <vilib>:"WPI_CANTalonSRX_ConfigBrakeCoast.vi"("Brake / Coast Mode"=w108, "CAN Talon SRX Ref"=w111) -> ("CAN Talon SRX Ref"=w76:T44)  [unwired: 8 in, 1 out]
  n99 = call <vilib>:"WPI_CANTalonSRX_ConfigBrakeCoast.vi"("Brake / Coast Mode"=w108, "CAN Talon SRX Ref"=w107) -> ("CAN Talon SRX Ref"=w73:T44)  [unwired: 8 in, 1 out]
  n100 = call <vilib>:"WPI_CANTalonSRX_ConfigStatusFrameRate.vi"("CAN Talon SRX Ref"=w25, "Talon SRX Status Frame"=WPI_CANTalonSRX_StatusFrame."General Status Frame", "Frame Rate Ms"=u32 200) -> ("CAN Talon SRX Ref"=w24:T44)  [unwired: 12 in]
  n101 = call <vilib>:"WPI_CANTalonSRX_SetReference.vi"("Feedback Reference"=WPI_CANTalonSRX_APIFeedbackSelect."CTR Magnetic Enc (Relative)", "CAN Talon SRX Ref"=w76) -> ("CAN Talon SRX Ref"=w75:T44)  [unwired: 8 in, 1 out]
  n102 = call <vilib>:"WPI_CANTalonSRX_ConfigStatusFrameRate.vi"("CAN Talon SRX Ref"=w48, "Talon SRX Status Frame"=WPI_CANTalonSRX_StatusFrame."General Status Frame", "Frame Rate Ms"=u32 200) -> ("CAN Talon SRX Ref"=w49:T44)  [unwired: 12 in]
  n103 = call <vilib>:"WPI_CANTalonSRX_ConfigStatusFrameRate.vi"("CAN Talon SRX Ref"=w66, "Talon SRX Status Frame"=WPI_CANTalonSRX_StatusFrame."General Status Frame", "Frame Rate Ms"=u32 200) -> ("CAN Talon SRX Ref"=w65:T44)  [unwired: 12 in]
  n104 = call <vilib>:"WPI_CANTalonSRX_SetReference.vi"("Reverse Feedback Sensor"=TRUE, "Feedback Reference"=WPI_CANTalonSRX_APIFeedbackSelect."CTR Magnetic Enc (Relative)", "CAN Talon SRX Ref"=w73) -> ("CAN Talon SRX Ref"=w72:T44)  [unwired: 7 in, 1 out]
  n105 = call <vilib>:"WPI_MotorControlRefNum Registry Set.vi"("refnum name"="Shooter Right", "MotorControlDevRef"=w75) -> ("MotorControlDevRef"=w67:T44)  [unwired: 8 in, 1 out]
  n106 = call <vilib>:"WPI_MotorControlRefNum Registry Set.vi"("refnum name"="Shooter Left", "MotorControlDevRef"=w72) -> ("MotorControlDevRef"=w70:T44)  [unwired: 8 in, 1 out]
  n107 = call <vilib>:"WPI_MotorControlRefNum Registry Set.vi"("refnum name"="Drivetrain Right", "MotorControlDevRef"=w24) -> ()  [unwired: 8 in, 2 out]
  n108 = global write "Robot Global Data.vi" "Autoshift Enabled?"(TRUE ("Autoshift Enabled?")) -> ()
  n109 = call <vilib>:"WPI_MotorControlSetOutput.vi"("Output"=0.0, "MotorControlDevRef"=w67) -> ()  [unwired: 7 in, 3 out]
  n110 = call <vilib>:"WPI_MotorControlRefNum Registry Set.vi"("refnum name"="Drivetrain Right 2", "MotorControlDevRef"=w49) -> ()  [unwired: 8 in, 2 out]
  n111 = call <vilib>:"WPI_MotorControlRefNum Registry Set.vi"("refnum name"="Drivetrain Right 1", "MotorControlDevRef"=w65) -> ()  [unwired: 8 in, 2 out]
  n112 = call <vilib>:"WPI_MotorControlSetOutput.vi"("Output"=0.0, "MotorControlDevRef"=w70) -> ()  [unwired: 7 in, 3 out]
  n113 = disable-structure shown="Enabled" {
    frame Disabled {
      n114 = call-poly <vilib>:"WPI_MotorControlOpen.vi"("Device Number"=u8 5) -> ("MotorControlDeviceRef"=w236:T44)  [unwired: 9 in, 1 out]
      n115 = call "624ClearTalonSettings.vi"("CAN Talon SRX Ref Out"=w236) -> ("CAN Talon SRX Ref Out 2"=w235:T44)  [unwired: 10 in]
      n116 = call-poly <vilib>:"WPI_MotorControlOpen.vi"("Invert"=TRUE, "Master Device Number"=u8 5, "Device Number"=u8 6, "Control Mode"=WPI_CANTalonSRX_APIControlMode."Slave") -> ("MotorControlDeviceRef"=w231:T44)  [unwired: 6 in, 1 out]
      n117 = call <vilib>:"WPI_CANTalonSRX_ConfigBrakeCoast.vi"("Brake / Coast Mode"=WPI_CANTalonSRX_BrakeOverride."Override to Coast", "CAN Talon SRX Ref"=w235) -> ("CAN Talon SRX Ref"=w234:T44)  [unwired: 8 in, 1 out]
      n118 = call "624ClearTalonSettings.vi"("CAN Talon SRX Ref Out"=w231) -> ()  [unwired: 10 in, 1 out]
      n119 = call <vilib>:"WPI_MotorControlRefNum Registry Set.vi"("refnum name"="Trigger", "MotorControlDevRef"=w234) -> ()  [unwired: 8 in, 2 out]
    }
    frame Enabled {
      n120 = call-poly <vilib>:"WPI_MotorControlOpen.vi"("PWM Channel"=FPGA_DIOPWMChannel."PWM 9") -> ("MotorControlDeviceRef"=w241:T44)  [unwired: 9 in, 1 out]
      n121 = call-poly <vilib>:"WPI_MotorControlOpen.vi"("PWM Channel"=FPGA_DIOPWMChannel."PWM 8") -> ("MotorControlDeviceRef"=w240:T44)  [unwired: 9 in, 1 out]
      n122 = call <vilib>:"WPI_MotorControlRefNum Registry Set.vi"("refnum name"="Trigger Right", "MotorControlDevRef"=w240) -> ()  [unwired: 8 in, 2 out]
      n123 = call <vilib>:"WPI_MotorControlRefNum Registry Set.vi"("refnum name"="Trigger Left", "MotorControlDevRef"=w241) -> ()  [unwired: 8 in, 2 out]
    }
  }
  n124 = disable-structure shown="Disabled" {
    frame Disabled {
      # "Climb"
      n125 = call-poly <vilib>:"WPI_MotorControlOpen.vi"("PWM Channel"=FPGA_DIOPWMChannel."PWM 4") -> ("MotorControlDeviceRef"=w245:T44)  [unwired: 9 in, 1 out]
      n126 = call <vilib>:"WPI_MotorControlRefNum Registry Set.vi"("refnum name"="Extender", "MotorControlDevRef"=w245) -> ()  [unwired: 8 in, 2 out]
    }
    frame Enabled {
    }
  }
  n127 = call <vilib>:"WPI_AnalogOutputOpen.vi"("AO Channel"=WPI_AnalogOutputChannel."AO MXP 0") -> ("AODeviceRef"=w4:T52)  [unwired: 9 in, 1 out]
  n128 = call <vilib>:"WPI_AnalogOutputOpen.vi"("AO Channel"=WPI_AnalogOutputChannel."AO MXP 1") -> ("AODeviceRef"=w7:T52)  [unwired: 9 in, 1 out]
  n129 = call <vilib>:"WPI_AnalogOutputRefNum Registry Set.vi"("refnum name"="Multiplexer", "AODeviceRef"=w4) -> ()  [unwired: 8 in, 2 out]
  n130 = call <vilib>:"WPI_AnalogOutputRefNum Registry Set.vi"("refnum name"="Status", "AODeviceRef"=w7) -> ()  [unwired: 8 in, 2 out]
  n131 = call <vilib>:"WPI_DigitalInputOpen.vi"("DIO Channel"=FPGA_DIOChannel."DIO 8") -> ("error out"=w101:errorcluster, "DigitalInputDevRef"=w100:T31)  [unwired: 9 in]
  n132 = call <vilib>:"WPI_DigitalInputRefNum Registry Set.vi"("error in (no error)"=w101, "refnum name"="Trigger Ball Detector", "DigitalInputDevRef"=w100) -> ()  [unwired: 7 in, 2 out]
  n133 = disable-structure shown="Disabled" {
    frame Disabled {
      n134 = call <vilib>:"WPI_DigitalOutputOpen.vi"("DIO Channel"=FPGA_DIOChannel."DIO 7") -> ("DigitalOutputDevRef"=w249:T53)  [unwired: 9 in, 1 out]
      n135 = call <vilib>:"WPI_DigitalOutputOpen.vi"("DIO Channel"=FPGA_DIOChannel."DIO 8") -> ("DigitalOutputDevRef"=w252:T53)  [unwired: 9 in, 1 out]
      n136 = call <vilib>:"WPI_DigitalOutputOpen.vi"("DIO Channel"=FPGA_DIOChannel."DIO 9") -> ("DigitalOutputDevRef"=w255:T53)  [unwired: 9 in, 1 out]
      n137 = call <vilib>:"WPI_DigitalOutputRefNum Registry Set.vi"("refnum name"="State 3", "DigitalOutputDevRef"=w249) -> ()  [unwired: 8 in, 2 out]
      n138 = call <vilib>:"WPI_DigitalOutputRefNum Registry Set.vi"("refnum name"="State 2", "DigitalOutputDevRef"=w252) -> ()  [unwired: 8 in, 2 out]
      n139 = call <vilib>:"WPI_DigitalOutputRefNum Registry Set.vi"("refnum name"="State 1", "DigitalOutputDevRef"=w255) -> ()  [unwired: 8 in, 2 out]
    }
    frame Enabled {
    }
  }
  n140 = call-poly <vilib>:"WPI_MotorControlOpen.vi"("PWM Channel"=FPGA_DIOPWMChannel."PWM 7") -> ("MotorControlDeviceRef"=w97:T44)  [unwired: 9 in, 1 out]
  n141 = call-poly <vilib>:"WPI_MotorControlOpen.vi"("Device Number"=u8 11) -> ("MotorControlDeviceRef"=w128:T44)  [unwired: 9 in, 1 out]
  n142 = call-poly <vilib>:"WPI_MotorControlOpen.vi"("Device Number"=u8 5) -> ("MotorControlDeviceRef"=w118:T44)  [unwired: 9 in, 1 out]
  n143 = call <vilib>:"WPI_MotorControlRefNum Registry Set.vi"("refnum name"="Intake Motor", "MotorControlDevRef"=w97) -> ()  [unwired: 8 in, 2 out]
  n144 = call <vilib>:"WPI_PotentiometerOpen.vi"("Analog Channel"=FPGA_AIChannel."AI 1") -> ("PotDevRef"=w124:T54)  [unwired: 9 in, 1 out]
  n145 = call "624ClearTalonSettings.vi"("CAN Talon SRX Ref Out"=w128) -> ("CAN Talon SRX Ref Out 2"=w129:T44)  [unwired: 10 in]
  n146 = call "624ClearTalonSettings.vi"("CAN Talon SRX Ref Out"=w118) -> ("CAN Talon SRX Ref Out 2"=w119:T44)  [unwired: 10 in]
  n147 = call <vilib>:"WPI_CANTalonSRX_ConfigBrakeCoast.vi"("Brake / Coast Mode"=WPI_CANTalonSRX_BrakeOverride."Override to Brake", "CAN Talon SRX Ref"=w119) -> ("CAN Talon SRX Ref"=w120:T44)  [unwired: 8 in, 1 out]
  n148 = call <vilib>:"WPI_PotentiometerRefNum Registry Set.vi"("refnum name"="Shooter String Pot", "PotDevRef"=w124) -> ()  [unwired: 8 in, 2 out]
  n149 = call <vilib>:"WPI_CANTalonSRX_ConfigBrakeCoast.vi"("Brake / Coast Mode"=WPI_CANTalonSRX_BrakeOverride."Override to Brake", "CAN Talon SRX Ref"=w129) -> ("CAN Talon SRX Ref"=w130:T44)  [unwired: 8 in, 1 out]
  n150 = call <vilib>:"WPI_MotorControlRefNum Registry Set.vi"("refnum name"="Intake Rotation", "MotorControlDevRef"=w130) -> ()  [unwired: 8 in, 2 out]
  n151 = call <vilib>:"WPI_MotorControlRefNum Registry Set.vi"("refnum name"="Angle Motor", "MotorControlDevRef"=w120) -> ()  [unwired: 8 in, 2 out]
  "error out" <- "error in"
